vi "MainUI.vi"() -> ()   [LabVIEW 2014]
uses:
  eng/trunk/ni/cRIO Master Files/Controls/StateMachineTypeDef.ctl
  eng/trunk/ni/cRIO Master Files/Controls/LogState.ctl
  <userlib>/ELL/EventLog/EventLog.lvclass
  <userlib>/ELL/EventLog/Initialize_CSV.vi
  eng/trunk/ni/cRIO Master Files/Controls/StringSelector.ctl
  eng/trunk/ni/cRIO Master Files/Controls/SystemControl.ctl
  eng/trunk/ni/cRIO Master Files/Controls/EnergyStorageStringData.ctl
  eng/trunk/ni/cRIO Master Files/Controls/NamedError.ctl
  eng/trunk/ni/cRIO Master Files/Controls/EnergyStorageSystemData.ctl
  Controls/FPGAData.ctl
  eng/trunk/ni/cRIO Master Files/Controls/PowerConversionData.ctl
panel:
  out "ES String Data":T1[](array[typedef])
  out "Voltage Difference":sgl
  out "Waveform Chart":T2(graph)
  out "Thermocouple Temperature":T3(graph)
  out "Temps":T4
  out "Module Indicators":T5
  out "Temp Data":T6
  out "BB RT State":T7(ring)
  in  "Clear Fault":bool
  out "PC Data":T8
  out "FPGA Data":T9
  out "ES System Data":T10={"Voltage"=0.0, "Current"=0.0, "SOC Avg"=0.0, "Faults"=0, "Alarms"=0, "Number of Strings"=0, "Max Temp"=0, "Min Temp"=0, "Max Cell Voltage"=0.0, "Min Cell Voltage"=0.0, "Energy Capacity (kWh)"=0.0, "Energy Remaining (kWh)"=0.0, "SOC Min"=0.0, "SOC Max"=0.0, "ES Fault"=FALSE, "String Selector"=enum."3 Strings", "ES Com Fault"=FALSE}
  in  "Data In":T12={"Start"=FALSE, "Stop"=FALSE, "Power System Enable"=FALSE, "SSG Control"=FALSE, "Virtual Inertia"=FALSE, "Manual Current"=FALSE, "Discharge"=FALSE, "Spot Generation"=FALSE, "Charge Control"=FALSE, "Watchdog"=FALSE, "ComAp Fault"=FALSE, "Clear Gen Faults"=FALSE, "Clear PV Faults"=FALSE, "Clear System Faults"=FALSE, "Clear PC Faults"=FALSE, "Clear ES Faults"=FALSE, "Clear Watchdog Faults"=FALSE, "PS V Setpoint"=0.0, "Manual Current"=0.0, "CC V Setpoint"=0.0, "Gen Capacity"=0.0, "Gen Reserve"=0.0, "VI gain P"=0.0, "CC gain P"=0.0, "Nom Hz"=0.0, "Spot Gen Op Value"=50.0, "CC gain I"=0.0, "CC Charge"=100.0, "CC Discharge"=-100.0, "Discharge Current"=-25.0, "Sign Of Life"=FALSE, "Reverse Rotation"=FALSE, "String Selector"=enum."3 Strings"}
  out "Log Rate Data":T6
  out "Network Stream":T6
  out "Flush Events":T6
  out "Queue Data Log":T6
  out "Data Logger":T6
  out "Log State":T13=enum."Rotate Log"
  in  "Exit Button":bool
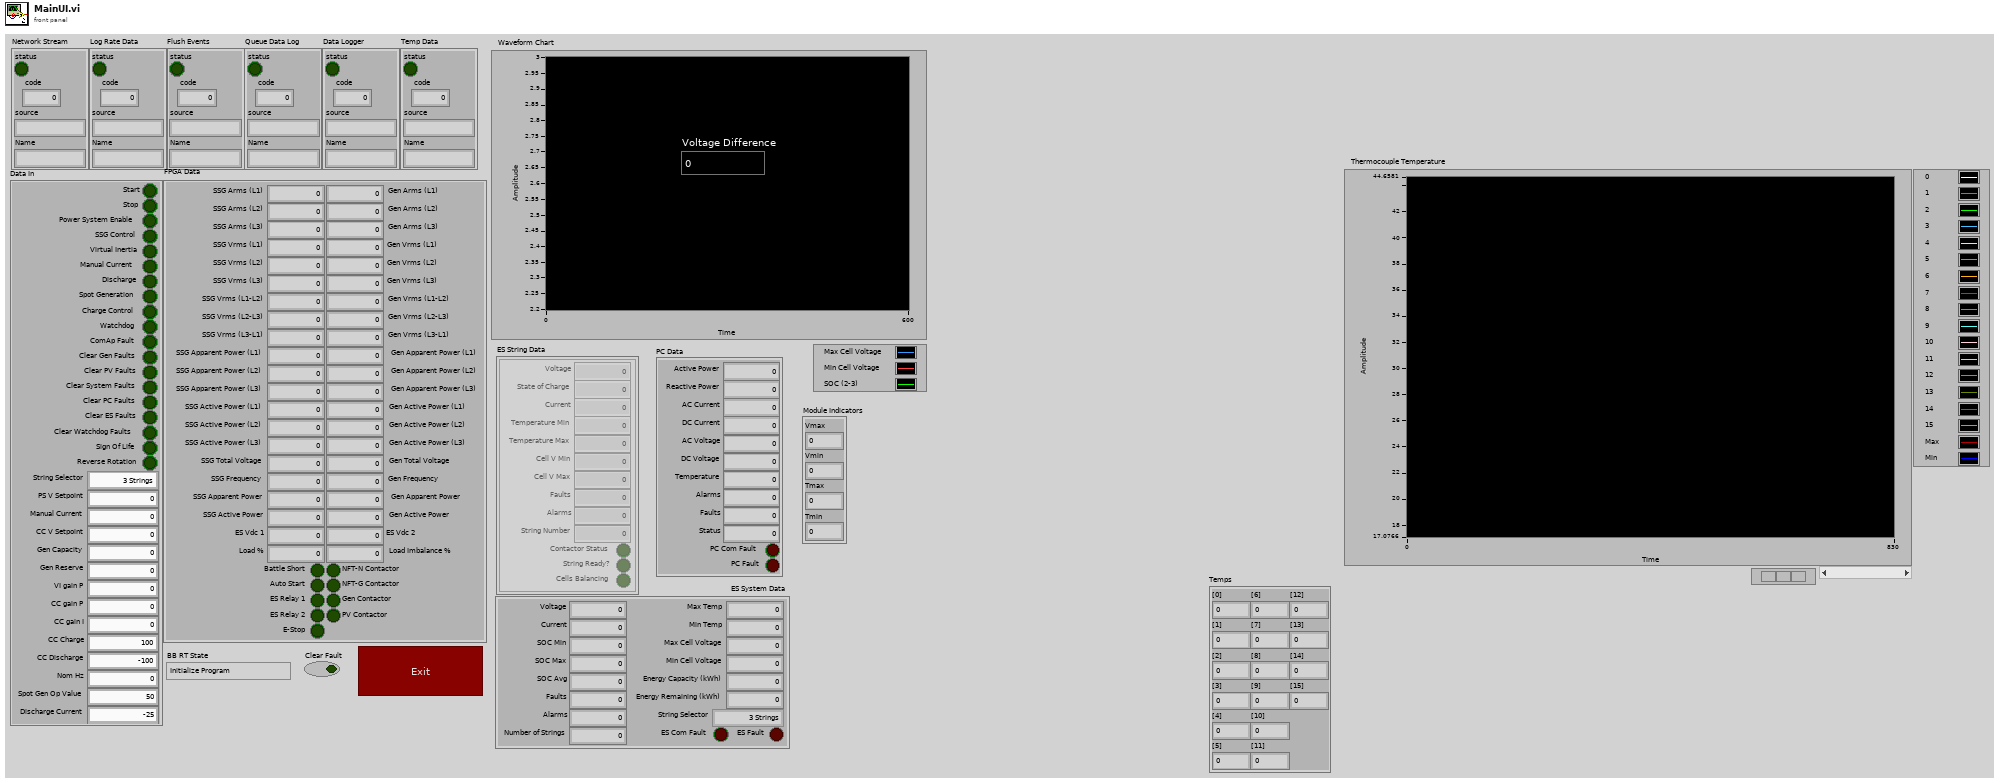
[diagram p1: front panel]
types:
  T1 = typedef "EnergyStorageStringData.ctl" = cluster{"Voltage":sgl, "State of Charge":sgl, "Current":sgl, "Temperature Min":i16, "Temperature Max":i16, "Faults":u16, "Alarms":u16, "String Number":u16, "Contactor Status":bool, "String Ready?":bool, "Cells Balancing":bool, "Cell V Max":dbl, "Cell V Min":dbl}
  T2 = cluster{"[0]":sgl, "[1]":sgl, "[2]":sgl, "[3]":sgl, "[4]":sgl, "[5]":sgl, "[6]":sgl, "[7]":sgl, "[8]":sgl}
  T3 = cluster{"[0]":dbl, "[1]":dbl, "[2]":dbl, "[3]":dbl, "[4]":dbl, "[5]":dbl, "[6]":dbl, "[7]":dbl, "[8]":dbl, "[9]":dbl, "[10]":dbl, "[11]":dbl, "[12]":dbl, "[13]":dbl, "[14]":dbl, "[15]":dbl, "[16]":dbl, "[17]":dbl}
  T4 = cluster{"[0]":dbl, "[1]":dbl, "[2]":dbl, "[3]":dbl, "[4]":dbl, "[5]":dbl, "[6]":dbl, "[7]":dbl, "[8]":dbl, "[9]":dbl, "[10]":dbl, "[11]":dbl, "[12]":dbl, "[13]":dbl, "[14]":dbl, "[15]":dbl}
  T5 = cluster{"Vmax":i16, "Vmin":i16, "Tmax":i16, "Tmin":i16}
  T6 = typedef "NamedError.ctl" = cluster{"status":bool, "code":i32, "source":string, "Name":string}
  T7 = enum16{"Initialize Program", "Big Boss Startup 1", "Big Boss Startup 2", "Big Boss Startup 3", "Big Boss Startup 4", "Big Boss Startup 5", "Big Boss Startup 6", "Shiner Startup 1", "Shiner Startup 2", "Shiner Startup 3", "Shiner Startup 4", "Shiner Startup 5", "Shiner Startup 6", "Shiner Startup 7", "Shiner Startup 8", "Shiner Startup 9", "Discharge", "Init Batteries", "Start s120", "enable batteries", "s120 Voltage Match", "Reset Batteries", "Wait for Event", "System Standby", "StandbyToRunning", "System Running", "SSG Enabled", "SpotGen Start", "SpotGen Charge", "SpotGen Desync", "SpotGen Discharge", "SpotGen Sync", "Peak Shave", "Charge Control", "Manual Current", "Inhibit Control", "Stop System", "uCap Start 1", "uCap Start 2", "uCap Start 3", "INVALID STATE"}
  T8 = typedef "PowerConversionData.ctl" = cluster{"Active Power":sgl, "Reactive Power":sgl, "AC Current":sgl, "DC Current":sgl, "AC Voltage":sgl, "DC Voltage":sgl, "Temperature":sgl, "Alarms":u16, "Faults":u16, "Status":u16, "PC Fault":bool, "PC Com Fault":bool}
  T9 = typedef "FPGAData.ctl" = cluster{"SSG Frequency":sgl, "SSG Total Voltage":dbl, "SSG Active Power":sgl, "SSG Apparent Power":sgl, "SSG Active Power (L1)":dbl, "SSG Active Power (L2)":dbl, "SSG Active Power (L3)":dbl, "SSG Apparent Power (L1)":dbl, "SSG Apparent Power (L2)":dbl, "SSG Apparent Power (L3)":dbl, "SSG Vrms (L1-L2)":dbl, "SSG Vrms (L2-L3)":dbl, "SSG Vrms (L3-L1)":dbl, "SSG Vrms (L1)":dbl, "SSG Vrms (L2)":dbl, "SSG Vrms (L3)":dbl, "SSG Arms (L1)":dbl, "SSG Arms (L2)":dbl, "SSG Arms (L3)":dbl, "Gen Frequency":sgl, "Gen Total Voltage":dbl, "Gen Active Power":sgl, "Gen Apparent Power":sgl, "Gen Active Power (L1)":dbl, "Gen Active Power (L2)":dbl, "Gen Active Power (L3)":dbl, "Gen Apparent Power (L1)":dbl, "Gen Apparent Power (L2)":dbl, "Gen Apparent Power (L3)":dbl, "Gen Vrms (L1-L2)":dbl, "Gen Vrms (L2-L3)":dbl, "Gen Vrms (L3-L1)":dbl, "Gen Vrms (L1)":dbl, "Gen Vrms (L2)":dbl, "Gen Vrms (L3)":dbl, "Gen Arms (L1)":dbl, "Gen Arms (L2)":dbl, "Gen Arms (L3)":dbl, "ES Vdc 1":sgl, "ES Vdc 2":sgl, "Load %":sgl, "Load Imbalance %":sgl, "E-Stop":bool, "Battle Short":bool, "Auto Start":bool, "Gen Contactor":bool, "ES Relay 1":bool, "ES Relay 2":bool, "NFT-N Contactor":bool, "NFT-G Contactor ":bool, "PV Contactor":bool}
  T10 = typedef "EnergyStorageSystemData.ctl" = cluster{"Voltage":sgl, "Current":sgl, "SOC Avg":sgl, "Faults":u16, "Alarms":u16, "Number of Strings":u16, "Max Temp":i16, "Min Temp":i16, "Max Cell Voltage":sgl, "Min Cell Voltage":sgl, "Energy Capacity (kWh)":sgl, "Energy Remaining (kWh)":sgl, "SOC Min":sgl, "SOC Max":sgl, "ES Fault":bool, "String Selector":T11, "ES Com Fault":bool}
  T11 = typedef "StringSelector.ctl" = enum16{"1 String (1)", "1 String (2)", "1 String (3)", "2 Strings (1 2)", "2 Strings (2 3)", "2 Strings (1 3)", "3 Strings"}
  T12 = typedef "SystemControl.ctl" = cluster{"Start":bool, "Stop":bool, "Power System Enable":bool, "SSG Control":bool, "Virtual Inertia":bool, "Manual Current":bool, "Discharge":bool, "Spot Generation":bool, "Charge Control":bool, "Watchdog":bool, "ComAp Fault":bool, "Clear Gen Faults":bool, "Clear PV Faults":bool, "Clear System Faults":bool, "Clear PC Faults":bool, "Clear ES Faults":bool, "Clear Watchdog Faults":bool, "PS V Setpoint":dbl, "Manual Current":dbl, "CC V Setpoint":dbl, "Gen Capacity":dbl, "Gen Reserve":dbl, "VI gain P":dbl, "CC gain P":dbl, "Nom Hz":dbl, "Spot Gen Op Value":dbl, "CC gain I":dbl, "CC Charge":dbl, "CC Discharge":dbl, "Discharge Current":dbl, "Sign Of Life":bool, "Reverse Rotation":bool, "String Selector":T11}
  T13 = typedef "LogState.ctl" = enum16{"Remove Null Data", "Rotate Log", "Log Data", "Wait", "Close File", "Open File"}
  T14 = typedef "StateMachineTypeDef.ctl" = enum16{"Idle", "Initialize", "Alarm Clicked", "go to Set Points", "go to Diagnostics", "go to Histogram", "go to Main", "go to Metering", "Enable Charge Control", "Enable External Control", "Enable Manual Current", "Enable Discharge", "Enable Virtual Inertia", "Start System", "Stop System", "Shutdown", "Error"}
  T15 = cluster{"SSG Frequency":sgl, "SSG Total Voltage":dbl, "SSG Active Power":sgl, "SSG Apparent Power":sgl, "SSG Active Power (L1)":dbl, "SSG Active Power (L2)":dbl, "SSG Active Power (L3)":dbl, "SSG Apparent Power (L1)":dbl, "SSG Apparent Power (L2)":dbl, "SSG Apparent Power (L3)":dbl, "SSG Vrms (L1-L2)":dbl, "SSG Vrms (L2-L3)":dbl, "SSG Vrms (L3-L1)":dbl, "SSG Vrms (L1)":dbl, "SSG Vrms (L2)":dbl, "SSG Vrms (L3)":dbl, "SSG Arms (L1)":dbl, "SSG Arms (L2)":dbl, "SSG Arms (L3)":dbl, "Gen Frequency":sgl, "Gen Total Voltage":dbl, "Gen Active Power":sgl, "Gen Apparent Power":sgl, "Gen Active Power (L1)":dbl, "Gen Active Power (L2)":dbl, "Gen Active Power (L3)":dbl, "Gen Apparent Power (L1)":dbl, "Gen Apparent Power (L2)":dbl, "Gen Apparent Power (L3)":dbl, "Gen Vrms (L1-L2)":dbl, "Gen Vrms (L2-L3)":dbl, "Gen Vrms (L3-L1)":dbl, "Gen Vrms (L1)":dbl, "Gen Vrms (L2)":dbl, "Gen Vrms (L3)":dbl, "Gen Arms (L1)":dbl, "Gen Arms (L2)":dbl, "Gen Arms (L3)":dbl, "ES Vdc 1":sgl, "ES Vdc 2":sgl, "Load %":sgl, "Load Imbalance %":sgl, "E-Stop":bool, "Battle Short":bool, "Auto Start":bool, "Gen Contactor":bool, "ES Relay 1":bool, "ES Relay 2":bool, "NFT-N Contactor":bool, "NFT-G Contactor ":bool, "PV Contactor":bool}
  T16 = typedef "StringSelector.ctl" = enum16{"1 String (1)", "1 String (2)", "1 String (3)", "2 Strings (1, 2)", "2 Strings (2, 3)", "2 Strings (1, 3)", "3 Strings"}
  T17 = cluster{"Voltage":sgl, "Current":sgl, "SOC Avg":sgl, "Faults":u16, "Alarms":u16, "Number of Strings":u16, "Max Temp":i16, "Min Temp":i16, "Max Cell Voltage":sgl, "Min Cell Voltage":sgl, "Energy Capacity (kWh)":sgl, "Energy Remaining (kWh)":sgl, "SOC Min":sgl, "SOC Max":sgl, "ES Fault":bool, "String Selector":T16}
  T18 = cluster{"Active Power":sgl, "Reactive Power":sgl, "AC Current":sgl, "DC Current":sgl, "AC Voltage":sgl, "DC Voltage":sgl, "Temperature":sgl, "Alarms":u16, "Faults":u16, "Status":u16, "PC Fault":bool, "PC Com Fault":bool}
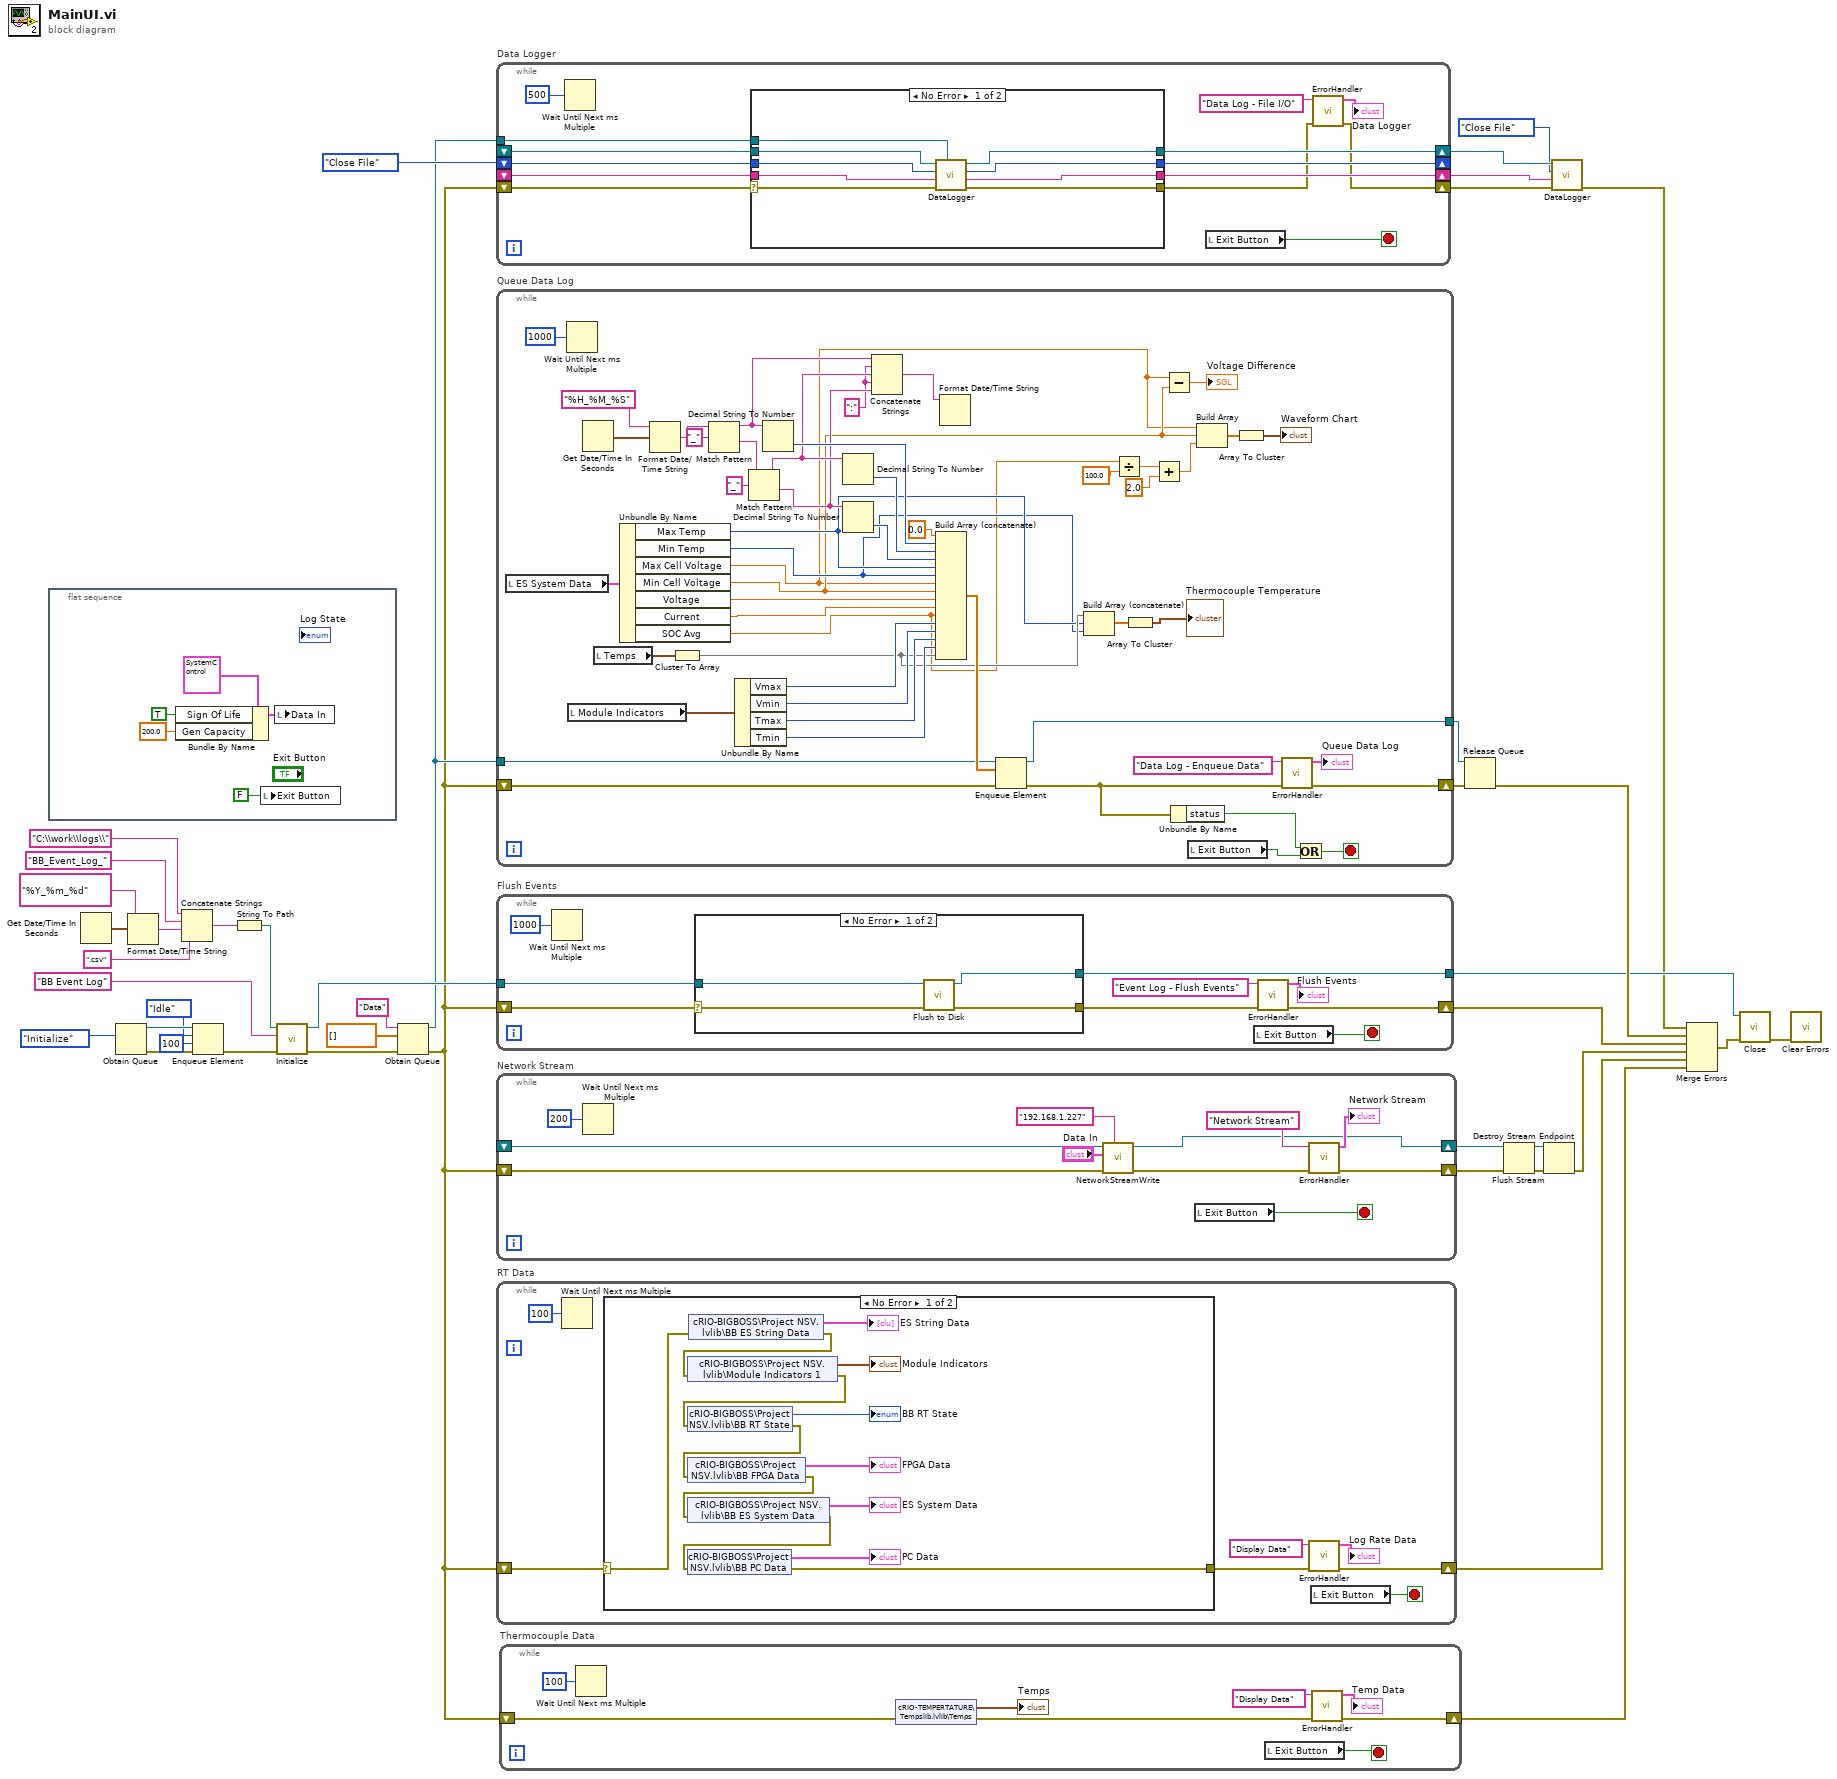
[diagram p0: block diagram]
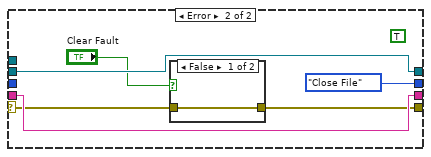
[diagram p2: hidden frame]
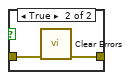
[diagram p3: hidden frame]
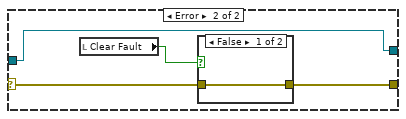
[diagram p4: hidden frame]
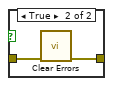
[diagram p5: hidden frame]
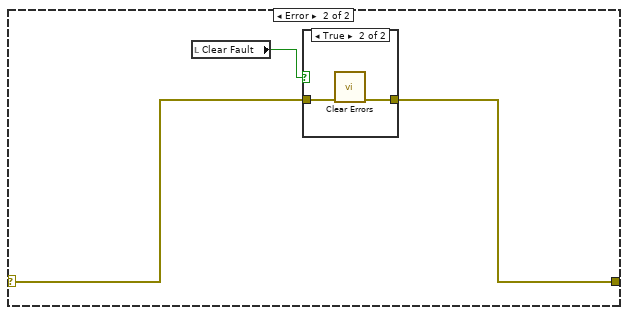
[diagram p6: hidden frame]
diagram:
  n1 = flat-sequence {
    frame #0 {
      n2 = Bundle By Name(cluster=T12 {"Start"=FALSE, "Stop"=FALSE, "Power System Enable"=FALSE, "SSG Control"=FALSE, "Virtual Inertia"=FALSE, "Manual Current"=FALSE, "Discharge"=FALSE, "Spot Generation"=FALSE, "Charge Control"=FALSE, "Watchdog"=FALSE, "ComAp Fault"=FALSE, "Clear Gen Faults"=FALSE, "Clear PV Faults"=FALSE, "Clear System Faults"=FALSE, "Clear PC Faults"=FALSE, "Clear ES Faults"=FALSE, "Clear Watchdog Faults"=FALSE, "PS V Setpoint"=0.0, "Manual Current"=0.0, "CC V Setpoint"=0.0, "Gen Capacity"=0.0, "Gen Reserve"=0.0, "VI gain P"=0.0, "CC gain P"=0.0, "Nom Hz"=0.0, "Spot Gen Op Value"=50.0, "CC gain I"=0.0, "CC Charge"=100.0, "CC Discharge"=-100.0, "Discharge Current"=-25.0, "Sign Of Life"=FALSE, "Reverse Rotation"=FALSE, "String Selector"=enum."3 Strings"} ("Data In"), "Sign Of Life"=TRUE, "Gen Capacity"=200.0) -> (w44:T12)
      n3 = local write "Exit Button"(FALSE ("Stop Button")) -> ()
      n4 = local write "Data In"(w44) -> ()
    }
  }
  n5 = Get Date/Time In Seconds() -> (seconds since 1Jan1904=w30:timestamp)
  n6 = Obtain Queue(element data type=StateMachineTypeDef."Initialize") -> (queue out=w39:refnum<queue>, error out=w40:errorcluster)  [unwired: 4 in, 1 out]
  n7 = Format Date/Time String(time format string (%c)="%Y_%m_%d", seconds (now)=w30) -> (date/time string=w29:string)  [unwired: 1 in]
  n8 = Concatenate Strings("C:\\work\\logs\\" ("string"), "BB_Event_Log_" ("string"), w29, ".csv" ("string")) -> (w28:string)
  n9 = Enqueue Element(queue=w39, element=StateMachineTypeDef."Idle", timeout in ms (-1)=100, error in (no error)=w40) -> (error out=w21:errorcluster)  [unwired: 2 out]
  n10 = String To Path(string=w28) -> (path=w27:path)
  n11 = call-poly <userlib>:"Initialize.vi"("error in (no error)"=w21, "Description"="BB Event Log", "Path"=w27) -> ("error out"=w20:errorcluster, "EventLog ref"=w13:refnum<class "EventLog.lvclass">)  [unwired: 7 in]
  n12 = Obtain Queue(name (unnamed)="Data", element data type=dbl[] [] ("appended array"), error in (no error)=w20) -> (queue out=w10:refnum<queue>, error out=w7:errorcluster)  [unwired: 2 in, 1 out]
  n13 = while "Data Logger" {
    shift-right: [w55] -> w2
    shift-left: _ -> [w54]
    shift-right: [w48] -> w5
    shift-left: w7 -> [w53]
    shift-right: [w56] -> _
    shift-left: LogState."Close File" ("Log State") -> [w57]
    shift-right: [w58] -> w3
    shift-left: _ -> [w59]
    tunnel: w10 -> [w47]
    stop <- w52 stop-if-true
    n14 = Wait Until Next ms Multiple(millisecond multiple=u32 500 ("milliseconds to wait")) -> ()  [unwired: 1 out]
    n15 = case shown="No Error" w53 {
      selector: w53 -> [w63 w71]
      tunnel: w59 -> [w65 w73]
      tunnel: [w64 w73] -> w58
      tunnel: w57 -> [w67 _]
      tunnel: [w62 w72] -> w51
      tunnel: [w66 LogState."Close File" ("Log State Out")] -> w56
      tunnel: [w68 w74] -> w55
      tunnel: w54 -> [w69 w74]
      tunnel: w47 -> [w61 _]
      frame No Error {
        n16 = call "DataLogger.vi"("Queue In"=w61, "Error In"=w63, "String In"=w65, "Log State In"=w67, "TDMS File In"=w69) -> ("Error Out"=w62:errorcluster, "String Out"=w64:string, "Log State Out"=w66:T13, "TDMS File Out"=w68:refnum<k34>)  [unwired: 1 in, 1 out]
      }
      frame Error {
        (unwired) TRUE ("Log Event? Out")
        n17 = case shown="False" "Clear Fault" {
          tunnel: w71 -> [w76 w78]
          tunnel: [w76 w77] -> w72
          frame False {
          }
          frame True {
            n18 = call <vilib>:"Clear Errors.vi"("error in (no error)"=w78) -> ("error out"=w77:errorcluster)  [unwired: 5 in, 1 out]
          }
        }
      }
    }
    n19 = local read "Exit Button"() -> (w52:bool)
    n20 = call "ErrorHandler.vi"("Error In"=w51, "Name"="Data Log - File I/O") -> ("Error Out"=w48:errorcluster, "Named Error Out"=→"Data Logger":T6)  [unwired: 6 in]
  }
  n21 = while "Queue Data Log" {
    shift-right: [w120] -> w15
    shift-left: w7 -> [w127]
    tunnel: w10 -> [w119]
    tunnel: [w106] -> w8
    stop <- w126 stop-if-true
    w97 = ":" ("string")
    n22 = local read "ES System Data"() -> (w109:T10)
    n23 = Wait Until Next ms Multiple(millisecond multiple=u32 1000 ("milliseconds to wait")) -> ()  [unwired: 1 out]
    n24 = local read "Module Indicators"() -> (w105:T5)
    n25 = Get Date/Time In Seconds() -> (seconds since 1Jan1904=w118:timestamp)
    n26 = local read "Temps"() -> (w94:T4)
    n27 = Unbundle By Name(w109) -> ("Max Temp"=w92:i16, "Min Temp"=w91:i16, "Max Cell Voltage"=w79:sgl, "Min Cell Voltage"=w80:sgl, "Voltage"=w108:sgl, "Current"=w107:sgl, "SOC Avg"=w81:sgl)
    n28 = Format Date/Time String(time format string (%c)="%H_%M_%S", seconds (now)=w118) -> (date/time string=w116:string)  [unwired: 1 in]
    n29 = Cluster To Array(cluster=w94) -> (array=w93:dbl[])
    n30 = Match Pattern(string=w116, regular expression="_") -> (before substring=w100:string, after substring=w113:string)  [unwired: 1 in, 2 out]
    n31 = Unbundle By Name(w105) -> ("Vmax"=w104:i16, "Vmin"=w103:i16, "Tmax"=w102:i16, "Tmin"=w101:i16)
    n32 = Match Pattern(string=w113, regular expression="_") -> (before substring=w99:string, after substring=w98:string)  [unwired: 1 in, 2 out]
    n33 = Decimal String To Number(string=w100) -> (number=w111:i32)  [unwired: 2 in, 1 out]
    n34 = Decimal String To Number(string=w99) -> (number=w112:i32)  [unwired: 2 in, 1 out]
    n35 = Decimal String To Number(string=w98) -> (number=w110:i32)  [unwired: 2 in, 1 out]
    n36 = Concatenate Strings(w100, w97, w99, w97, w98) -> (w96:string)
    n37 = Build Array (concatenate)(0.0 ("element"), w111, w112, w110, w92, w91, w79, w80, w108, w107, w81, w104, w103, w102, w101, w93) -> (w128:dbl[])
    n38 = Format Date/Time String(time format string (%c)=w96) -> ()  [unwired: 2 in, 1 out]
    n39 = Enqueue Element(queue=w119, element=w128, error in (no error)=w127) -> (queue out=w106:refnum<queue>, error out=w123:errorcluster)  [unwired: 1 in, 1 out]
    n40 = Build Array (concatenate)(w93, w92, w91) -> (w90:dbl[])
    n41 = Divide(x=w81, y=sgl 100.0) -> (x/y=w87:sgl)
    n42 = Array To Cluster(array=w90) -> (cluster=→"Thermocouple Temperature":T3)
    n43 = Add(x=w87, y=sgl 2.0) -> (x+y=w85:sgl)
    n44 = Subtract(x=w79, y=w80) -> (x-y=→"Voltage Difference":sgl)
    n45 = Unbundle By Name(w123) -> ("status"=w124:bool)
    n46 = local read "Exit Button"() -> (w125:bool)
    n47 = Build Array(w79, w80, w85) -> (w84:sgl[])
    n48 = Array To Cluster(array=w84) -> (cluster=→"Waveform Chart":T2)
    n49 = call "ErrorHandler.vi"("Error In"=w123, "Name"="Data Log - Enqueue Data") -> ("Error Out"=w120:errorcluster, "Named Error Out"=→"Queue Data Log":T6)  [unwired: 6 in]
    n50 = Or(x=w124, y=w125) -> (x .or. y?=w126:bool)
  }
  n51 = while "Flush Events" {
    tunnel: w13 -> [w138]
    shift-right: [w132] -> w12
    shift-left: w7 -> [w136]
    tunnel: [w130] -> w9
    stop <- w131 stop-if-true
    n52 = Wait Until Next ms Multiple(millisecond multiple=u32 1000 ("milliseconds to wait")) -> ()  [unwired: 1 out]
    n53 = case shown="No Error" w136 {
      selector: w136 -> [w140 w146]
      tunnel: [w142 w145] -> w135
      tunnel: w138 -> [w141 w143]
      tunnel: [w139 w143] -> w130
      frame No Error {
        n54 = call <userlib>:"Flush to Disk.vi"("error in (no error)"=w140, "EventLog ref"=w141) -> ("error out"=w142:errorcluster, "EventLog ref"=w139:refnum<class "EventLog.lvclass">)  [unwired: 8 in]
      }
      frame Error {
        n55 = local read "Clear Fault"() -> (w144:bool)
        n56 = case shown="False" w144 {
          tunnel: w146 -> [w147 w149]
          tunnel: [w147 w148] -> w145
          frame False {
          }
          frame True {
            n57 = call <vilib>:"Clear Errors.vi"("error in (no error)"=w149) -> ("error out"=w148:errorcluster)  [unwired: 5 in, 1 out]
          }
        }
      }
    }
    n58 = local read "Exit Button"() -> (w131:bool)
    n59 = call "ErrorHandler.vi"("Error In"=w135, "Name"="Event Log - Flush Events") -> ("Error Out"=w132:errorcluster, "Named Error Out"=→"Flush Events":T6)  [unwired: 6 in]
  }
  n60 = while "Network Stream" {
    shift-right: [w152] -> w16
    shift-left: _ -> [w157]
    shift-right: [w153] -> w17
    shift-left: w7 -> [w158]
    stop <- w159 stop-if-true
    n61 = Wait Until Next ms Multiple(millisecond multiple=u32 200 ("milliseconds to wait")) -> ()  [unwired: 1 out]
    n62 = call "NetworkStreamWrite.vi"("Ip Address"="192.168.1.227", "Error In"=w158, "Data In"="Data In", "Network Stream Ref In"=w157) -> ("Error Out"=w156:errorcluster, "Network Stream Ref Out"=w152:refnum<k21>)  [unwired: 5 in, 1 out]
    n63 = local read "Exit Button"() -> (w159:bool)
    n64 = call "ErrorHandler.vi"("Error In"=w156, "Name"="Network Stream") -> ("Error Out"=w153:errorcluster, "Named Error Out"=→"Network Stream":T6)  [unwired: 6 in]
  }
  n65 = while "RT Data" {
    shift-right: [w161] -> w18
    shift-left: w7 -> [w166]
    stop <- w165 stop-if-true
    n66 = Wait Until Next ms Multiple(millisecond multiple=u32 100 ("milliseconds to wait")) -> ()  [unwired: 1 out]
    n67 = case shown="No Error" w166 {
      selector: w166 -> [w170 w183]
      tunnel: [w177 w182] -> w164
      frame No Error {
        n68 = shared-variable "cRIO-BIGBOSS\\Project NSV.lvlib\\BB ES String Data"(error in=w170) -> (→"ES String Data":T1[], error out=w169:errorcluster)
        n69 = shared-variable "cRIO-BIGBOSS\\Project NSV.lvlib\\Module Indicators 1"(error in=w169) -> (→"Module Indicators":T5, error out=w172:errorcluster)
        n70 = shared-variable "cRIO-BIGBOSS\\Project NSV.lvlib\\BB RT State"(error in=w172) -> (→"BB RT State":T7, error out=w174:errorcluster)
        n71 = shared-variable "cRIO-BIGBOSS\\Project NSV.lvlib\\BB FPGA Data"(error in=w174) -> (→"FPGA Data":T15, error out=w175:errorcluster)
        n72 = shared-variable "cRIO-BIGBOSS\\Project NSV.lvlib\\BB ES System Data"(error in=w175) -> (→"ES System Data":T17, error out=w176:errorcluster)
        n73 = shared-variable "cRIO-BIGBOSS\\Project NSV.lvlib\\BB PC Data"(error in=w176) -> (→"PC Data":T18, error out=w177:errorcluster)
      }
      frame Error {
        n74 = local read "Clear Fault"() -> (w181:bool)
        n75 = case shown="True" w181 {
          tunnel: w183 -> [w184 w186]
          tunnel: [w184 w185] -> w182
          frame False {
          }
          frame True {
            n76 = call <vilib>:"Clear Errors.vi"("error in (no error)"=w186) -> ("error out"=w185:errorcluster)  [unwired: 5 in, 1 out]
          }
        }
      }
    }
    n77 = call "ErrorHandler.vi"("Error In"=w164, "Name"="Display Data") -> ("Error Out"=w161:errorcluster, "Named Error Out"=→"Log Rate Data":T6)  [unwired: 6 in]
    n78 = local read "Exit Button"() -> (w165:bool)
  }
  n79 = while "Thermocouple Data" {
    shift-right: [w190] -> w6
    shift-left: w7 -> [w192]
    stop <- w188 stop-if-true
    n80 = Wait Until Next ms Multiple(millisecond multiple=u32 100 ("milliseconds to wait")) -> ()  [unwired: 1 out]
    n81 = shared-variable "cRIO-TEMPERTATURE\\Tempslib.lvlib\\Temps"(error in=w192) -> (→"Temps":T4, error out=w191:errorcluster)
    n82 = local read "Exit Button"() -> (w188:bool)
    n83 = call "ErrorHandler.vi"("Error In"=w191, "Name"="Display Data") -> ("Error Out"=w190:errorcluster, "Named Error Out"=→"Temp Data":T6)  [unwired: 6 in]
  }
  n84 = Release Queue(queue=w8, error in (no error)=w15) -> (error out=w22:errorcluster)  [unwired: 1 in, 2 out]
  n85 = Flush Stream(8:w17, 11:w16) -> (0:w37:errorcluster, 3:w36:refnum<k21>)  [unwired: 2 in, 1 out]
  n86 = Destroy Stream Endpoint(8:w37, 11:w36) -> (0:w34:errorcluster)
  n87 = call "DataLogger.vi"("Error In"=w5, "String In"=w3, "Log State In"=LogState."Close File", "TDMS File In"=w2) -> ("Error Out"=w4:errorcluster)  [unwired: 2 in, 4 out]
  n88 = Merge Errors(w4, w22, w12, w34, w18, w6) -> (w11:errorcluster)
  n89 = call <userlib>:"Close.vi"("error in (no error)"=w11, "EventLog ref"=w9) -> ("error out"=w19:errorcluster)  [unwired: 9 in]
  n90 = call <vilib>:"Clear Errors.vi"("error in (no error)"=w19) -> ()  [unwired: 5 in, 2 out]
